vi "DESTROY UE 2.vi"(8 "error in (no error)":errorcluster, 11 "GRAFICAR_SEÑAL_ACTUALIZABLE in":refnum<class "GRAFICAR_SEÑAL_ACTUALIZABLE.lvclass">) -> (0 "error out":errorcluster, 3 "GRAFICAR_SEÑAL_ACTUALIZABLE out":refnum<class "GRAFICAR_SEÑAL_ACTUALIZABLE.lvclass">)   [LabVIEW 2019, in "GRAFICAR_SEÑAL_ACTUALIZABLE.lvlib" / "GRAFICAR_SEÑAL_ACTUALIZABLE.lvclass"]
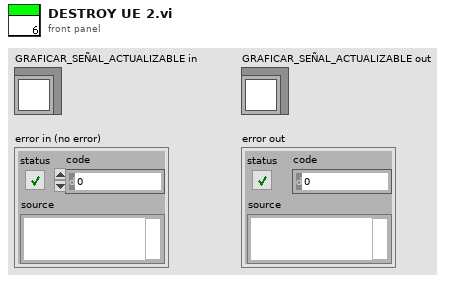
[diagram p1: front panel]
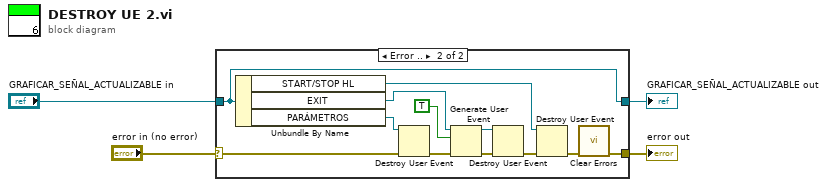
[diagram p0: block diagram]
diagram:
  n1 = case shown="Error .." "error in (no error)" {
    selector: "error in (no error)" -> [w6 w8]
    tunnel: "GRAFICAR_SEÑAL_ACTUALIZABLE in" -> [w5 w10]
    tunnel: [w6 w11] -> w3
    tunnel: [w5 w10] -> w4
    frame No Error {
    }
    frame Error {
      n2 = Unbundle By Name(w10) -> ("START/STOP HL"=w15:refnum<user-event>, "EXIT"=w18:refnum<user-event>, "PARÁMETROS"=w9:refnum<user-event>)
      n3 = Destroy User Event(user event=w9, error in=w8) -> (error out=w7:errorcluster)
      n4 = Generate User Event(user event=w18, event data cluster=TRUE ("event data"), error in=w7) -> (user event out=w16:refnum<user-event>, error out=w17:errorcluster)  [unwired: 1 in]
      n5 = Destroy User Event(user event=w16, error in=w17) -> (error out=w14:errorcluster)
      n6 = Destroy User Event(user event=w15, error in=w14) -> (error out=w12:errorcluster)
      n7 = call <vilib>:"Clear Errors.vi"("error in (no error)"=w12) -> ("error out"=w11:errorcluster)  [unwired: 5 in, 1 out]
    }
  }
  "GRAFICAR_SEÑAL_ACTUALIZABLE out" <- w4
  "error out" <- w3
